vi "通用文件传输.vi"(4 "目的文件路径（使用对话框）":path=path "C:/Users/Administrator.2W964MZOGI5HE3B/Desktop/105256rhad11pc5553vz5e.png", 5 "字符串":string) -> ()   [LabVIEW 2016, in "数据传输系统.lvlib" / "自动更新.lvlib" / "TCP文件传输系统.lvlib" / "TCP接收文件.lvlib"]
panel:
  out "长度 2":i32
  out "错误输出 2":errorcluster caption="错误输出"
  out "长度":i32
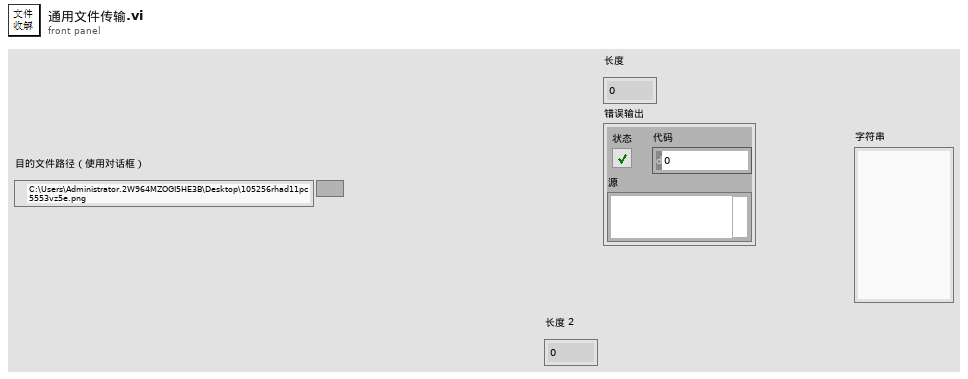
[diagram p1: front panel]
types:
  T1 = enum16{"big-endian, network order", "native, host order", "little-endian"}
  T2 = enum16{"open", "replace", "create", "open or create", "replace or create", "replace or create with confirmation"}
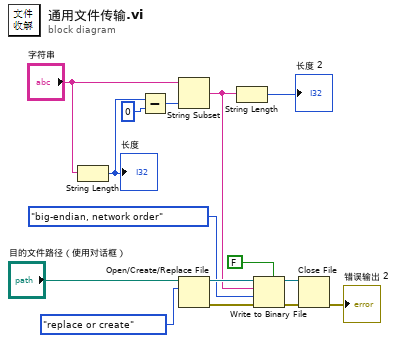
[diagram p0: block diagram]
diagram:
  n1 = String Length(string="字符串") -> (length=w6:i32)
  "长度" <- w6
  n2 = Subtract(x=w6, y=0) -> (x-y=w4:i32)
  n3 = String Subset(string="字符串", length (rest)=w4) -> (substring=w3:string)  [unwired: 1 in]
  n4 = Open/Create/Replace File(file path (use dialog)="目的文件路径（使用对话框）", operation (0:open)=T2."replace or create" ("操作(0:open)")) -> (refnum out=w13:refnum<file>, error out=w12:errorcluster)  [unwired: 4 in, 1 out]
  n5 = String Length(string=w3) -> (length=→"长度 2":i32)
  n6 = Write to Binary File(file (use dialog)=w13, data=w3, error in=w12, 5:FALSE ("预置数组或字符串大小？(T)"), 9:T1."big-endian, network order" ("字节顺序(0:big-endian, network order)")) -> (refnum out=w8:refnum<file>, error out=w11:errorcluster)  [unwired: 1 in, 1 out]
  n7 = Close File(refnum=w8, error in=w11) -> (error out=→"错误输出 2":errorcluster)  [unwired: 1 out]
